vi "SEA_9811_InitDynamicFPGA.vi"(7 "Run?":bool=TRUE, 8 "error in (no error)":errorcluster, 10 "FPGA resource name":T1 caption="RIO Device", 11 "Bitfile Path":path) -> (0 "error out":errorcluster, 3 "SEA9811_RT_data out":T2 {"Tx"."Tx Refs (Data,Trig)"."Data Reference" format="%.0x"})   [LabVIEW 2015]
uses:
  Typdefs/SEA9811_RT_data_cluster.ctl
  <userlib>/_FPGA Interface Advanced Tools/FPGA Interface Base/FPGA Interface Base.lvclass
  Typdefs/FPGA ref.ctl
  Typdefs/channel.ctl
  Typdefs/received word.ctl
  Typdefs/SEA9811_FPGA_FP_Addresses.ctl
  <vilib>/NI Veristand/Custom Device API/Block Data Reference.ctl
  <vilib>/NI Veristand/Custom Device API/Data Reference.ctl
  <vilib>/userdefined/High Color/nirio_resource_hc.ctl
  <userlib>/_FPGA Interface Advanced Tools/FPGA Interface Wrapper/TypeDefs/Open Attribute.ctl
  <vilib>/rvi/DataTransferAndStorage/Container/Common/niFpgaDataTypeControl.ctl
  <userlib>/_FPGA Interface Advanced Tools/FPGA Interface Base/FPGA Interface Base.lvclass/FPGA Interface Base.ctl
  <vilib>/Utility/error.llb/Error Cluster From Error Code.vi
  <userlib>/_FPGA Interface Advanced Tools/FPGA Interface Wrapper/FPGA Interface Wrapper.lvlib
  <vilib>/NI VeriStand/Custom Device API/Custom Device API.lvlib
  <vilib>/NI VeriStand/Custom Device Tools/Custom Device Utility Library/Custom Device Utility Library.lvlib
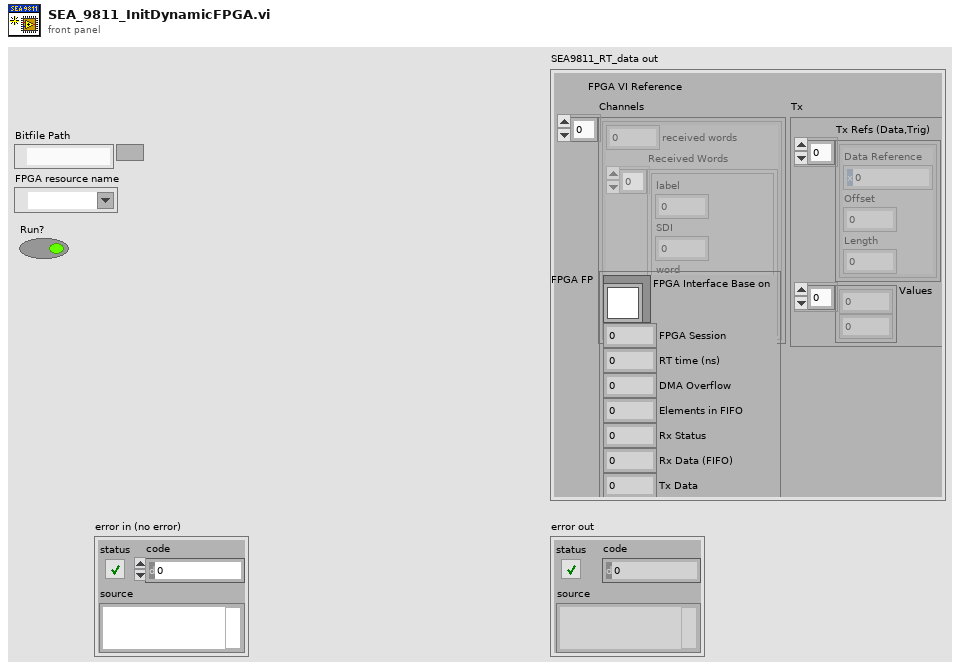
[diagram p1: front panel]
types:
  T1 = typedef "nirio_resource_hc.ctl" = tag
  T2 = typedef "SEA9811_RT_data_cluster.ctl" = cluster{"FPGA VI Reference":T3, "Channels":T4[], "FPGA FP":T6, "Tx":cluster{"Tx Refs (Data,Trig)":T7[], "Values":dbl[]}}
  T3 = typedef "FPGA ref.ctl" = refnum<k20>
  T4 = typedef "channel.ctl" = cluster{"received words":u32, "Received Words":T5[]}
  T5 = typedef "received word.ctl" = cluster{"label":u8, "SDI":u8, "word":u32, "timestamp":dbl}
  T6 = typedef "SEA9811_FPGA_FP_Addresses.ctl" = cluster{"FPGA Interface Base on":refnum<class "FPGA Interface Base.lvclass">, "FPGA Session":u32, "RT time (ns)":u32, "DMA Overflow":u32, "Elements in FIFO":u32, "Rx Status":u32, "Rx Data (FIFO)":u32, "Tx Data":u32, "Transmit Data":u32}
  T7 = typedef "Custom Device API.lvlib/Block Data Reference.ctl" = cluster{"Data Reference":T8, "Offset":u64, "Length":u64}
  T8 = typedef "Custom Device API.lvlib/Data Reference.ctl" = i32
  T9 = typedef "niFpgaDataTypeControl.ctl" = enum32{"Boolean", "I8", "I16", "I32", "I64", "U8", "U16", "U32", "U64", "FXP", "CustomControl", "SGL"}
  T10 = typedef "FPGA Interface Wrapper.lvlib/Open Attribute.ctl" = enum32{"Run (Default)", "No Run"}
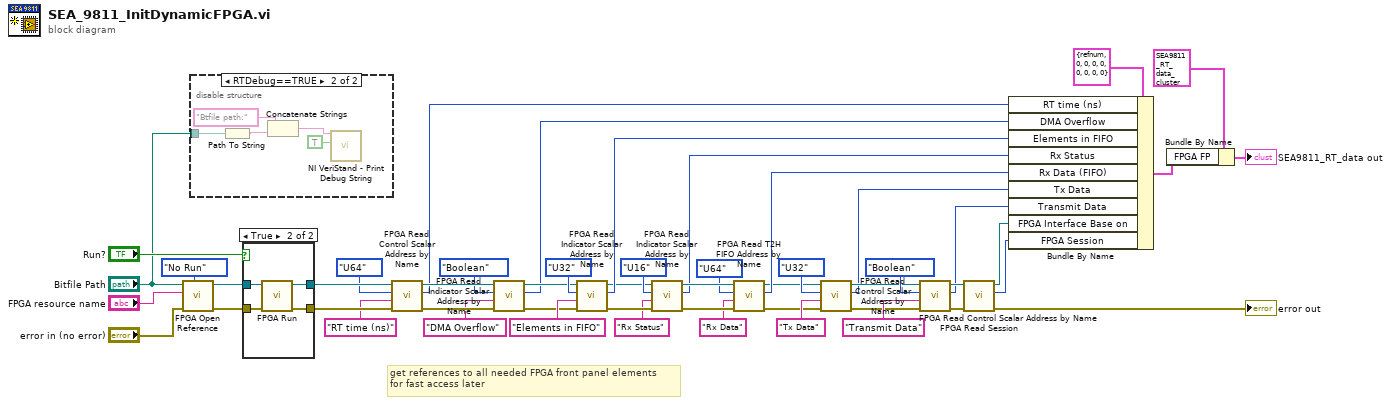
[diagram p0: block diagram]
diagram:
  # "get references to all needed FPGA front panel elements\nfor fast access later"
  n1 = call <userlib>:"FPGA Open Reference.vi"("Run?"=Open_Attribute."No Run", "error in (no error)"="error in (no error)", "FPGA Resource"="FPGA resource name", "Bitfile Path"="Bitfile Path") -> ("error out"=w49:errorcluster, "FPGA Session"=w48:refnum<class "FPGA Interface Base.lvclass">)  [unwired: 6 in]
  n2 = disable-structure shown="RTDebug==TRUE" {
    disable-tunnel: "Bitfile Path" -> [_ w55]
    frame condition #0 (active) {
    }
    frame condition #1 {
      n3 = Path To String(path=w55) -> (string=w53:string)
      n4 = Concatenate Strings("Btfile path:" ("string"), w53) -> (w52:string)
      n5 = call <vilib>:"NI VeriStand - Print Debug String.vi"("Add to log file? (T)"=TRUE, "Message"=w52) -> ()  [unwired: 9 in, 1 out]
    }
  }
  n6 = case shown="True" "Run?" {
    tunnel: w48 -> [w57 w59]
    tunnel: w49 -> [w56 w58]
    tunnel: [w56 w61] -> w43
    tunnel: [w57 w60] -> w44
    frame False {
    }
    frame True {
      n7 = call <userlib>:"FPGA Run.vi"("error in (no error)"=w58, "FPGA Session In"=w59) -> ("error out"=w61:errorcluster, "FPGA Session Out"=w60:refnum<class "FPGA Interface Base.lvclass">)  [unwired: 8 in]
    }
  }
  n8 = call <userlib>:"FPGA Read Control Scalar Address by Name.vi"("error in (no error)"=w43, "Name"="RT time (ns)" ("Control"), "Data Type"=niFpgaDataTypeControl."U64", "FPGA Interface Base in"=w44) -> ("error out"=w38:errorcluster, "Address"=w18:u32, "FPGA Interface Base out"=w39:refnum<class "FPGA Interface Base.lvclass">)  [unwired: 4 in, 1 out]
  n9 = call <userlib>:"FPGA Read Indicator Scalar Address by Name.vi"("error in (no error)"=w38, "Name"="DMA Overflow" ("Control"), "Data Type"=niFpgaDataTypeControl."Boolean", "FPGA Interface Base in"=w39) -> ("error out"=w32:errorcluster, "Address"=w31:u32, "FPGA Interface Base out"=w33:refnum<class "FPGA Interface Base.lvclass">)  [unwired: 4 in, 1 out]
  n10 = call <userlib>:"FPGA Read Indicator Scalar Address by Name.vi"("error in (no error)"=w32, "Name"="Elements in FIFO" ("Control"), "Data Type"=niFpgaDataTypeControl."U32", "FPGA Interface Base in"=w33) -> ("error out"=w29:errorcluster, "Address"=w30:u32, "FPGA Interface Base out"=w26:refnum<class "FPGA Interface Base.lvclass">)  [unwired: 4 in, 1 out]
  n11 = call <userlib>:"FPGA Read Indicator Scalar Address by Name.vi"("Name"="Rx Status" ("Control"), "Data Type"=niFpgaDataTypeControl."U16", "FPGA Interface Base in"=w26) -> ("Address"=w24:u32, "FPGA Interface Base out"=w25:refnum<class "FPGA Interface Base.lvclass">)  [unwired: 5 in, 2 out]
  n12 = call <userlib>:"FPGA Read T2H FIFO Address by Name.vi"("error in (no error)"=w29, "Name"="Rx Data" ("Control"), "Data Type"=niFpgaDataTypeControl."U64", "FPGA Interface Base in"=w25) -> ("error out"=w11:errorcluster, "Address"=w21:u32, "FPGA Interface Base out"=w10:refnum<class "FPGA Interface Base.lvclass">)  [unwired: 4 in, 1 out]
  n13 = call <userlib>:"FPGA Read Control Scalar Address by Name.vi"("error in (no error)"=w11, "Name"="Tx Data" ("Control"), "Data Type"=niFpgaDataTypeControl."U32", "FPGA Interface Base in"=w10) -> ("error out"=w6:errorcluster, "Address"=w2:u32, "FPGA Interface Base out"=w7:refnum<class "FPGA Interface Base.lvclass">)  [unwired: 4 in, 1 out]
  n14 = call <userlib>:"FPGA Read Control Scalar Address by Name.vi"("error in (no error)"=w6, "Name"="Transmit Data" ("Control"), "Data Type"=niFpgaDataTypeControl."Boolean", "FPGA Interface Base in"=w7) -> ("error out"=w5:errorcluster, "Address"=w3:u32, "FPGA Interface Base out"=w4:refnum<class "FPGA Interface Base.lvclass">)  [unwired: 4 in, 1 out]
  n15 = call <userlib>:"FPGA Read Session.vi"("error in (no error)"=w5, "FPGA Interface Base in"=w4) -> ("error out"=→"error out":errorcluster, "FPGA Session"=w19:u32, "FPGA Interface Base out"=w20:refnum<class "FPGA Interface Base.lvclass">)  [unwired: 7 in]
  n16 = Bundle By Name(cluster=T6 {"FPGA Interface Base on"=refnum, "FPGA Session"=0, "RT time (ns)"=0, "DMA Overflow"=0, "Elements in FIFO"=0, "Rx Status"=0, "Rx Data (FIFO)"=0, "Tx Data"=0, "Transmit Data"=0} ("FPGA FP"), "RT time (ns)"=w18, "DMA Overflow"=w31, "Elements in FIFO"=w30, "Rx Status"=w24, "Rx Data (FIFO)"=w21, "Tx Data"=w2, "Transmit Data"=w3, "FPGA Interface Base on"=w20, "FPGA Session"=w19) -> (w14:T6)
  n17 = Bundle By Name(cluster=T2 {"FPGA VI Reference"=refnum, "Channels"=[], "FPGA FP"={"FPGA Interface Base on"=refnum, "FPGA Session"=0, "RT time (ns)"=0, "DMA Overflow"=0, "Elements in FIFO"=0, "Rx Status"=0, "Rx Data (FIFO)"=0, "Tx Data"=0, "Transmit Data"=0}, "Tx"={"Tx Refs (Data,Trig)"=[], "Values"=[]}} ("SEA9811_RT_data out"), "FPGA FP"=w14) -> (→"SEA9811_RT_data out":T2)
